vi "LUCS001RT_GPS_RS232_GetI32Data.vi"(1 "N-Bytes":u8[](array[numeric])=[96, 57, 252, 15, 42, 208, 229, 185, 4, 137, 9, 20, 84, 3, 3, 0, 255, 136, 3, 0, 136, 15, 0, 0, 223, 21, 0, 0, 116, 9] format="%02x", 3 "index":i32) -> (0 "I32":i32)   [LabVIEW 2020]
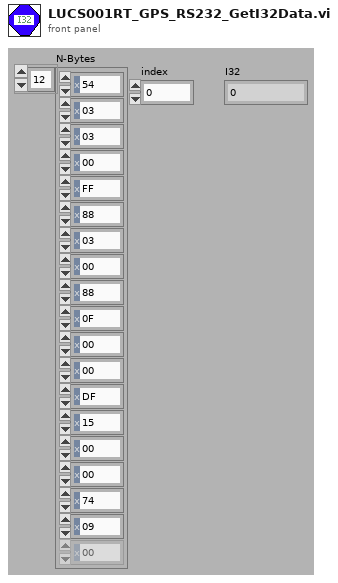
[diagram p1: front panel]
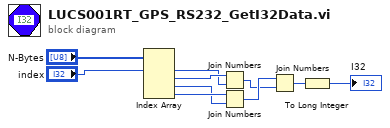
[diagram p0: block diagram]
diagram:
  n1 = Index Array(array="N-Bytes", index #1="index") -> (element #1=w5:u8, element #2=w6:u8, element #3=w7:u8, element #4=w8:u8)  [unwired: 3 in]
  n2 = Join Numbers(hi=w6, lo=w5) -> ((hi.lo)=w3:u16)
  n3 = Join Numbers(hi=w8, lo=w7) -> ((hi.lo)=w4:u16)
  n4 = Join Numbers(hi=w4, lo=w3) -> ((hi.lo)=w2:u32)
  n5 = To Long Integer(number=w2) -> (32bit integer=→"I32":i32)
